vi "MergeOverrideViWithMethod_V2.vi"(8 "error in":errorcluster, 10 "OverrideVIRef":refnum<vi>, 11 "ViRef":refnum<vi>) -> (0 "error out":errorcluster)   [LabVIEW 2020, in "ClassWriterNative.lvclass"]
uses:
  <resource>/Framework/Providers/Open_GDS/ClassProviders/Provider_LvNativeClass/ClassWriterNative_class/ClassWriterNative.lvclass
  <vilib>/Utility/miscctls.llb/LVPositionTypeDef.ctl
  <vilib>/addons/analyzer/_analyzerutils.llb/VIAnUtil Check Type If ErrClust.vi
  <vilib>/Utility/Data Type/NI_Data Type.lvlib
panel:
  out "Error-Indicator WiringRule":T1(ring)
  out "Error-Control WiringRule":T1(ring)
  out "Err-Indicator Index":i32
  out "Error-Control Index":i32
  out "DD_Indicator Index":i32
  out "DD-Control Index":i32
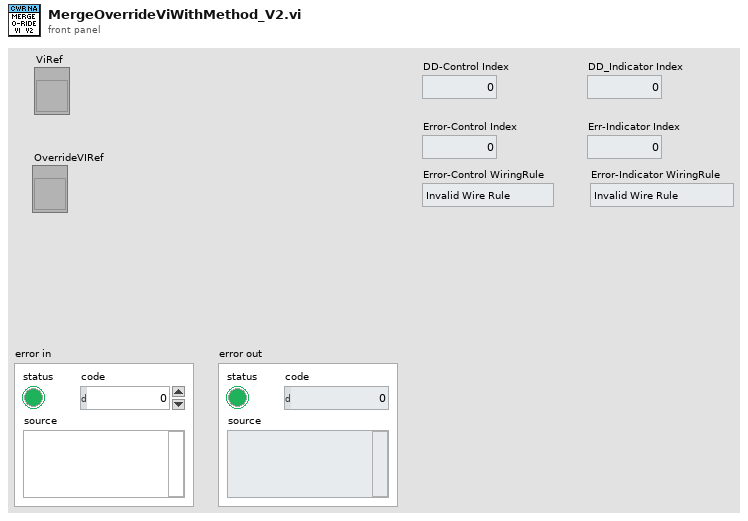
[diagram p1: front panel]
types:
  T1 = enum16{"Invalid Wire Rule", "Required", "Recommended", "Optional", "Dynamic Dispatch"}
  T2 = typedef "LVPositionTypeDef.ctl" = cluster{"Left":i32, "Top":i32}
  T3 = enum16{"Invalid Wire Rule", "Required", "Recommended", "Optional", "Dynamic Dispatch"}[]
  T4 = cluster{i32, refnum<vi>, "Wire Rule":enum16{"Invalid Wire Rule", "Required", "Recommended", "Optional", "Dynamic Dispatch"}, "Label.Text":string}
  T5 = typedef "LVRectTypeDef.ctl" = cluster{"Left":i16, "Top":i16, "Right":i16, "Bottom":i16}
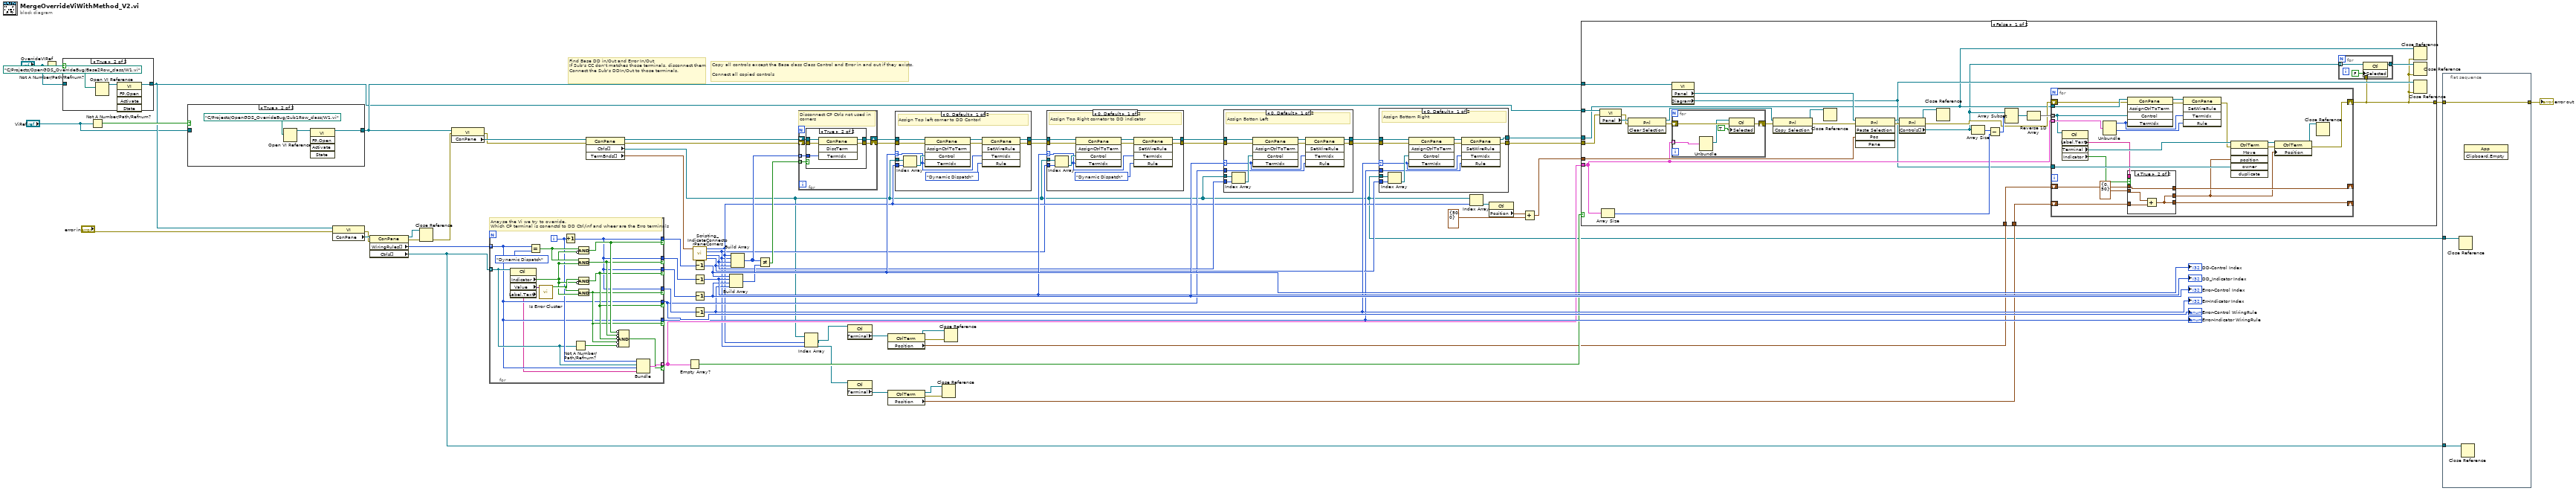
[diagram p0: block diagram]
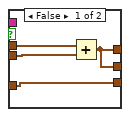
[diagram p4: hidden frame]
diagram:
  # "Find Base DD in/Out and Error In/Out\nIf Sub's CC don't matches those terminals, disconnect them\nConnect the Sub's DDIn/Out to those terminals."
  # "Copy all controls except the Base class Class Control and Error in and out if they exists.\n\nConnect all copied controls"
  n1 = Not A Number/Path/Refnum?(number/path/refnum="OverrideVIRef") -> (NaN/Path/Refnum?=w17:bool)
  n2 = case shown="True" w17 {
    tunnel: [w66 w67] -> w15
    tunnel: "OverrideVIRef" -> [w66 _]
    frame False {
    }
    frame True {
      n3 = Open VI Reference(vi path=path "C:/Projects/OpenGDS_OverrideBug/Base2Row_class/W1.vi") -> (vi reference=w68:refnum<vi>)  [unwired: 5 in, 1 out]
      n4 = invoke class="VI" method="FP.Open"(reference=w68) -> (reference out=w67:refnum<vi>)  [unwired: 4 in, 4 out]
    }
  }
  n5 = Not A Number/Path/Refnum?(number/path/refnum="ViRef") -> (NaN/Path/Refnum?=w16:bool)
  n6 = case shown="True" w16 {
    tunnel: [w70 w71] -> w65
    tunnel: "ViRef" -> [w70 _]
    frame False {
    }
    frame True {
      n7 = Open VI Reference(vi path=path "C:/Projects/OpenGDS_OverrideBug/Sub1Row_class/W1.vi") -> (vi reference=w72:refnum<vi>)  [unwired: 5 in, 1 out]
      n8 = invoke class="VI" method="FP.Open"(reference=w72) -> (reference out=w71:refnum<vi>)  [unwired: 4 in, 4 out]
    }
  }
  n9 = property class="VI"(reference=w15, error in="error in") -> (error out=w46:errorcluster, "ConPane"=w64:refnum<vi>)  [unwired: 1 out]
  n10 = property class="ConPane"(reference=w64, error in=w46) -> (reference out=w11:refnum<vi>, error out=w13:errorcluster, "WiringRules[]"=w63:T3, "Ctrls[]"=w9:refnum<vi>[])
  n11 = Close Reference(reference=w11, error in (no error)=w13) -> (error out=w12:errorcluster)
  n12 = property class="VI"(reference=w65, error in=w12) -> (error out=w47:errorcluster, "ConPane"=w57:refnum<vi>)  [unwired: 1 out]
  n13 = for {
    tunnel: w63 -> [w77] mode=indexing
    tunnel: [w80] -> w60 if=w85
    tunnel: w9 -> [w78] mode=indexing
    tunnel: [w80] -> w59 if=w84
    tunnel: [w80] -> w55 if=w83
    tunnel: [w80] -> w56 if=w82
    tunnel: [w77] -> w39 if=w83
    tunnel: [w77] -> w34 if=w82
    tunnel: [w76] -> w27 mode=indexing if=w75
    i -> [w79]
    # "Anayse the Vi we try to override.\nWhich CP terminal is conenctd to DD Ctrl/inf and wheer are the Erro terminals"
    n14 = property class="Ctl"(reference=w78) -> ("Indicator"=w86:bool, "Value"=w88:variant, "Label.Text"=w74:string)  [unwired: 1 in, 2 out]
    n15 = Equal?(x=w77, y=T1."Dynamic Dispatch") -> (x = y?=w89:bool)
    n16 = call <vilib>:"Is Error Cluster.vi"("variant"=w88) -> ("is error cluster?"=w87:bool)  [unwired: 9 in, 1 out]
    n17 = Increment(x=w79) -> (x+1=w80:i32)
    n18 = Not A Number/Path/Refnum?(number/path/refnum=w78) -> (NaN/Path/Refnum?=w81:bool)
    n19 = Compound Arithmetic op=AND(w89, invert w86) -> (w85:bool)
    n20 = Compound Arithmetic op=AND(w89, w86) -> (w84:bool)
    n21 = Compound Arithmetic op=AND(w87, invert w86) -> (w83:bool)
    n22 = Compound Arithmetic op=AND(w87, w86) -> (w82:bool)
    n23 = Compound Arithmetic op=AND(invert w85, invert w84, invert w83, invert w82, invert w81) -> (w75:bool)
    n24 = Bundle(w79, w78, "Wire Rule"=w77, "Label.Text"=w74) -> (w76:T4)  [unwired: 1 in]
  }
  "Error-Control WiringRule" <- w39
  "Error-Indicator WiringRule" <- w34
  n25 = property class="ConPane"(reference=w57, error in=w47) -> (reference out=w50:refnum<vi>, error out=w48:errorcluster, "Ctrls[]"=w3:refnum<vi>[], "TermBnds[]"=w58:T5[])
  n26 = Empty Array?(array=w27) -> (empty?=w26:bool)
  n27 = call <resource>:"Scripting_IndicateConnectorPaneCorners.vi"("TermBnds[]"=w58) -> ("RightLower"=w35:i32, "LeftLower"=w40:i32, "RightTop"=w24:i32, "LeftTop"=w25:i32)  [unwired: 7 in]
  n28 = Decrement(x=w60) -> (x-1=w54:i32)
  "DD-Control Index" <- w54
  n29 = Decrement(x=w59) -> (x-1=w53:i32)
  "DD_Indicator Index" <- w53
  n30 = Decrement(x=w55) -> (x-1=w41:i32)
  "Error-Control Index" <- w41
  n31 = Decrement(x=w56) -> (x-1=w36:i32)
  "Err-Indicator Index" <- w36
  n32 = Build Array(w54, w53, w41, w36) -> (w52:i32[])
  n33 = Build Array(w25, w24, w40, w35) -> (w49:i32[])
  n34 = Not Equal?(x=w49, y=w52) -> (x != y?=w51:bool[])
  n35 = for {
    shift-right: [w95] -> w61
    shift-left: w50 -> [w96]
    tunnel: w51 -> [w94] mode=indexing
    tunnel: w49 -> [w93] mode=indexing
    shift-right: [w91] -> w45
    shift-left: w48 -> [w92]
    # "Disconnect CP Ctrls not used in corners"
    n36 = case shown="True" w94 {
      tunnel: w96 -> [w97 w102]
      tunnel: [_ w101] -> w91
      tunnel: [w97 w100] -> w95
      tunnel: w93 -> [_ w99]
      tunnel: w92 -> [_ w98]
      frame False {
      }
      frame True {
        n37 = invoke class="ConPane" method="DiscTerm"(reference=w102, error in=w98, "TermIdx"=w99) -> (reference out=w100:refnum<vi>, error out=w101:errorcluster)  [unwired: 1 in, 2 out]
      }
    }
  }
  n38 = Index Array(array=w3, index #1=w25, index #2=w24) -> (element #1=w23:refnum<vi>, element #2=w20:refnum<vi>)
  n39 = property class="Ctl"(reference=w23) -> ("Terminal"=w22:refnum<vi>)  [unwired: 1 in, 2 out]
  n40 = property class="Ctl"(reference=w20) -> ("Terminal"=w21:refnum<vi>)  [unwired: 1 in, 2 out]
  n41 = property class="CtrlTerm"(reference=w22) -> (reference out=w6:refnum<vi>, error out=w7:errorcluster, "Position"=w19:T2)  [unwired: 1 in]
  n42 = property class="CtrlTerm"(reference=w21) -> (reference out=w4:refnum<vi>, error out=w5:errorcluster, "Position"=w18:T2)  [unwired: 1 in]
  n43 = case shown="0, Default" w54 {
    selector: w54 -> [w103 _]
    tunnel: w61 -> [w113 w115]
    tunnel: w3 -> [w112 _]
    tunnel: [w108 w115] -> w62
    tunnel: w25 -> [w107 _]
    tunnel: w45 -> [w106 w114]
    tunnel: [w104 w114] -> w44
    frame 0, Default {
      # "Assign Top left corner to DD Contorl"
      n44 = Index Array(array=w112, index=w107) -> (element=w111:refnum<vi>)
      n45 = invoke class="ConPane" method="AssignCtrlToTerm"(reference=w113, error in=w106, "Control"=w111, "TermIdx"=w103) -> (reference out=w110:refnum<vi>, error out=w105:errorcluster)  [unwired: 1 in, 3 out]
      n46 = invoke class="ConPane" method="SetWireRule"(reference=w110, error in=w105, "TermIdx"=w103, "Rule"=T1."Dynamic Dispatch" ("y")) -> (reference out=w108:refnum<vi>, error out=w104:errorcluster)  [unwired: 1 in, 3 out]
    }
    frame -1 {
    }
  }
  n47 = Close Reference(reference=w4, error in (no error)=w5) -> ()  [unwired: 1 out]
  n48 = Close Reference(reference=w6, error in (no error)=w7) -> ()  [unwired: 1 out]
  n49 = case shown="0, Default" w53 {
    selector: w53 -> [w116 _]
    tunnel: w62 -> [w126 w127]
    tunnel: w3 -> [w125 _]
    tunnel: w24 -> [w121 _]
    tunnel: w44 -> [w120 w128]
    tunnel: [w118 w128] -> w43
    tunnel: [w117 w127] -> w42
    frame 0, Default {
      # "Assign Top Right cornetor to DD indicator"
      n50 = Index Array(array=w125, index=w121) -> (element=w124:refnum<vi>)
      n51 = invoke class="ConPane" method="AssignCtrlToTerm"(reference=w126, error in=w120, "Control"=w124, "TermIdx"=w116) -> (reference out=w123:refnum<vi>, error out=w119:errorcluster)  [unwired: 1 in, 3 out]
      n52 = invoke class="ConPane" method="SetWireRule"(reference=w123, error in=w119, "TermIdx"=w116, "Rule"=T1."Dynamic Dispatch" ("y")) -> (reference out=w117:refnum<vi>, error out=w118:errorcluster)  [unwired: 1 in, 3 out]
    }
    frame -1 {
    }
  }
  n53 = case shown="0, Default" w41 {
    selector: w41 -> [w134 _]
    tunnel: w42 -> [w139 w141]
    tunnel: w3 -> [w138 _]
    tunnel: [w135 w141] -> w38
    tunnel: w40 -> [w133 _]
    tunnel: w43 -> [w132 w140]
    tunnel: [w130 w140] -> w37
    tunnel: w39 -> [w129 _]
    frame 0, Default {
      # "Assign Botton Left"
      n54 = Index Array(array=w138, index=w133) -> (element=w137:refnum<vi>)
      n55 = invoke class="ConPane" method="AssignCtrlToTerm"(reference=w139, error in=w132, "Control"=w137, "TermIdx"=w134) -> (reference out=w136:refnum<vi>, error out=w131:errorcluster)  [unwired: 1 in, 3 out]
      n56 = invoke class="ConPane" method="SetWireRule"(reference=w136, error in=w131, "TermIdx"=w134, "Rule"=w129) -> (reference out=w135:refnum<vi>, error out=w130:errorcluster)  [unwired: 1 in, 3 out]
    }
    frame -1 {
    }
  }
  n57 = case shown="0, Default" w36 {
    selector: w36 -> [w147 _]
    tunnel: w38 -> [w152 w154]
    tunnel: w3 -> [w151 _]
    tunnel: [w148 w154] -> w28
    tunnel: w35 -> [w146 _]
    tunnel: w37 -> [w145 w153]
    tunnel: [w143 w153] -> w33
    tunnel: w34 -> [w142 _]
    frame 0, Default {
      # "Assign Bottom Right"
      n58 = Index Array(array=w151, index=w146) -> (element=w150:refnum<vi>)
      n59 = invoke class="ConPane" method="AssignCtrlToTerm"(reference=w152, error in=w145, "Control"=w150, "TermIdx"=w147) -> (reference out=w149:refnum<vi>, error out=w144:errorcluster)  [unwired: 1 in, 3 out]
      n60 = invoke class="ConPane" method="SetWireRule"(reference=w149, error in=w144, "TermIdx"=w147, "Rule"=w142) -> (reference out=w148:refnum<vi>, error out=w143:errorcluster)  [unwired: 1 in, 3 out]
    }
    frame -1 {
    }
  }
  n61 = Index Array(array=w3, index=w25) -> (element=w32:refnum<vi>)
  n62 = property class="Ctl"(reference=w32) -> ("Position"=w31:T2)  [unwired: 1 in, 2 out]
  n63 = Add(x=w31, y=T2 {"Left"=50, "Top"=0}) -> (x+y=w30:T2)
  n64 = case shown="False" w26 {
    tunnel: w33 -> [w183 w223]
    tunnel: w65 -> [w176 _]
    tunnel: w15 -> [w175 _]
    tunnel: w30 -> [w173 _]
    tunnel: w28 -> [w158 _]
    tunnel: w27 -> [w166 _]
    tunnel: w19 -> [w165 _]
    tunnel: w18 -> [w164 _]
    tunnel: [w155 w223] -> w10
    frame False {
      n65 = property class="VI"(reference=w175, error in=w183) -> (error out=w181:errorcluster, "Panel"=w182:refnum<vi>)  [unwired: 1 out]
      n66 = Array Size(array=w166) -> (size(s)=w169:i32)
      n67 = invoke class="Pnl" method="Clear Selection"(reference=w182, error in=w181) -> (reference out=w177:refnum<vi>, error out=w180:errorcluster)  [unwired: 1 in, 1 out]
      n68 = property class="VI"(reference=w176) -> ("Panel"=w174:refnum<vi>, "Diagram"=w159:refnum<vi>)  [unwired: 1 in, 2 out]
      n69 = for {
        tunnel: w166 -> [w220] mode=indexing
        shift-right: [w218] -> w178
        shift-left: w180 -> [w221]
        n70 = Unbundle(w220) -> (w219:refnum<vi>)  [unwired: 3 out]
        n71 = property class="Ctl"(reference=w219, error in=w221, "Selected"=TRUE) -> (error out=w218:errorcluster)  [unwired: 1 out]
      }
      n72 = invoke class="Pnl" method="Copy Selection"(reference=w177, error in=w178) -> (reference out=w161:refnum<vi>, error out=w179:errorcluster)  [unwired: 1 in, 1 out]
      n73 = Close Reference(reference=w161) -> ()  [unwired: 1 in, 1 out]
      n74 = invoke class="Pnl" method="Paste Selection"(reference=w174, error in=w179, "Pos"=w173) -> (reference out=w172:refnum<vi>, error out=w171:errorcluster)  [unwired: 2 in, 3 out]
      n75 = property class="Pnl"(reference=w172, error in=w171) -> (reference out=w160:refnum<vi>, error out=w162:errorcluster, "Controls[]"=w157:refnum<vi>[])
      n76 = Close Reference(reference=w160) -> ()  [unwired: 1 in, 1 out]
      n77 = Array Size(array=w157) -> (size(s)=w170:i32)
      n78 = Subtract(x=w170, y=w169) -> (x-y=w168:i32)
      n79 = Array Subset(array=w157, index=w168) -> (w167:refnum<vi>[])  [unwired: 1 in]
      n80 = Reverse 1D Array(array=w167) -> (reversed array=w163:refnum<vi>[])
      n81 = for {
        tunnel: w158 -> [w208]
        tunnel: w166 -> [w207] mode=indexing
        tunnel: w163 -> [w203] mode=indexing
        tunnel: w159 -> [w199]
        shift-right: [w194] -> _
        shift-left: w165 -> [w197]
        shift-right: [w193] -> _
        shift-left: w164 -> [w196]
        shift-right: [w188] -> w155
        shift-left: w162 -> [w189]
        n82 = property class="Ctl"(reference=w203) -> ("Label.Text"=w190:string, "Terminal"=w201:refnum<vi>, "Indicator"=w198:bool)  [unwired: 1 in, 2 out]
        n83 = Unbundle(w207) -> (w206:i32, "Wire Rule"=w205:T1)  [unwired: 2 out]
        n84 = invoke class="ConPane" method="AssignCtrlToTerm"(reference=w208, error in=w189, "Control"=w203, "TermIdx"=w206) -> (reference out=w204:refnum<vi>, error out=w209:errorcluster)  [unwired: 1 in, 3 out]
        n85 = case shown="True" w198 {
          tunnel: w197 -> [w213 w217]
          tunnel: w196 -> [w211 w216]
          tunnel: T2 {"Left"=0, "Top"=50} ("y") -> [w212 w215]
          tunnel: [w210 w217] -> w194
          tunnel: [w211 w214] -> w193
          tunnel: [w210 w214] -> w191
          tunnel: w190 -> [_ _]
          frame False {
            n86 = Add(x=w213, y=w212) -> (x+y=w210:T2)
          }
          frame True {
            n87 = Add(x=w215, y=w216) -> (x+y=w214:T2)
          }
        }
        n88 = invoke class="ConPane" method="SetWireRule"(reference=w204, error in=w209, "TermIdx"=w206, "Rule"=w205) -> (error out=w192:errorcluster)  [unwired: 1 in, 4 out]
        n89 = invoke class="CtrlTerm" method="Move"(reference=w201, error in=w192, "position"=w191, "owner"=w199) -> (reference out=w200:refnum<vi>, error out=w202:errorcluster)  [unwired: 2 in, 4 out]
        n90 = property class="CtrlTerm"(reference=w200, error in=w202, "Position"=w191) -> (reference out=w187:refnum<vi>, error out=w188:errorcluster)
        n91 = Close Reference(reference=w187) -> ()  [unwired: 1 in, 1 out]
      }
      n92 = for {
        tunnel: w157 -> [w185] mode=indexing
        tunnel: [w184] -> w156
        tunnel: w155 -> [_]
        n93 = property class="Ctl"(reference=w185, "Selected"=FALSE) -> (reference out=w184:refnum<vi>)  [unwired: 1 in, 1 out]
      }
      n94 = Close Reference(reference=w158, error in (no error)=w155) -> ()  [unwired: 1 out]
      n95 = Close Reference(reference=w156, error in (no error)=w155) -> ()  [unwired: 1 out]
      n96 = Close Reference(reference=w159, error in (no error)=w155) -> ()  [unwired: 1 out]
    }
    frame True {
    }
  }
  n97 = flat-sequence {
    tunnel: w10 -> [w226]
    tunnel: [w226] -> w8
    tunnel: w9 -> [w225]
    tunnel: w3 -> [w224]
    frame #0 {
      n98 = Close Reference(reference=w224) -> ()  [unwired: 1 in, 1 out]
      n99 = Close Reference(reference=w225) -> ()  [unwired: 1 in, 1 out]
      n100 = invoke class="App" method="Clipboard.Empty"() -> ()  [unwired: 3 in, 3 out]
    }
  }
  "error out" <- w8
